vi "Receive Data From Aircraft.vi"(8 "error in (no error)":errorcluster) -> (0 "error out":errorcluster)   [LabVIEW 2014]
uses:
  Controls/Coms Driver Interface.ctl
  Telemetry/Controls/Telemetry Connection Type.ctl
  <vilib>/httpClient/ClientHandle.ctl
  Controls/Coms Driver State.ctl
  Application Support/Stop Button/SubVI/Get Stop Button Status.vi
  Web Services/DronePi Global Variables.vi
  Aircraft Information/Sub VI/Selected Aircraft/SubVI/Get Selected Aircraft.vi
  <vilib>/httpClient/LabVIEWHTTPClient.lvlib
panel:
  in  "Cluster":T1
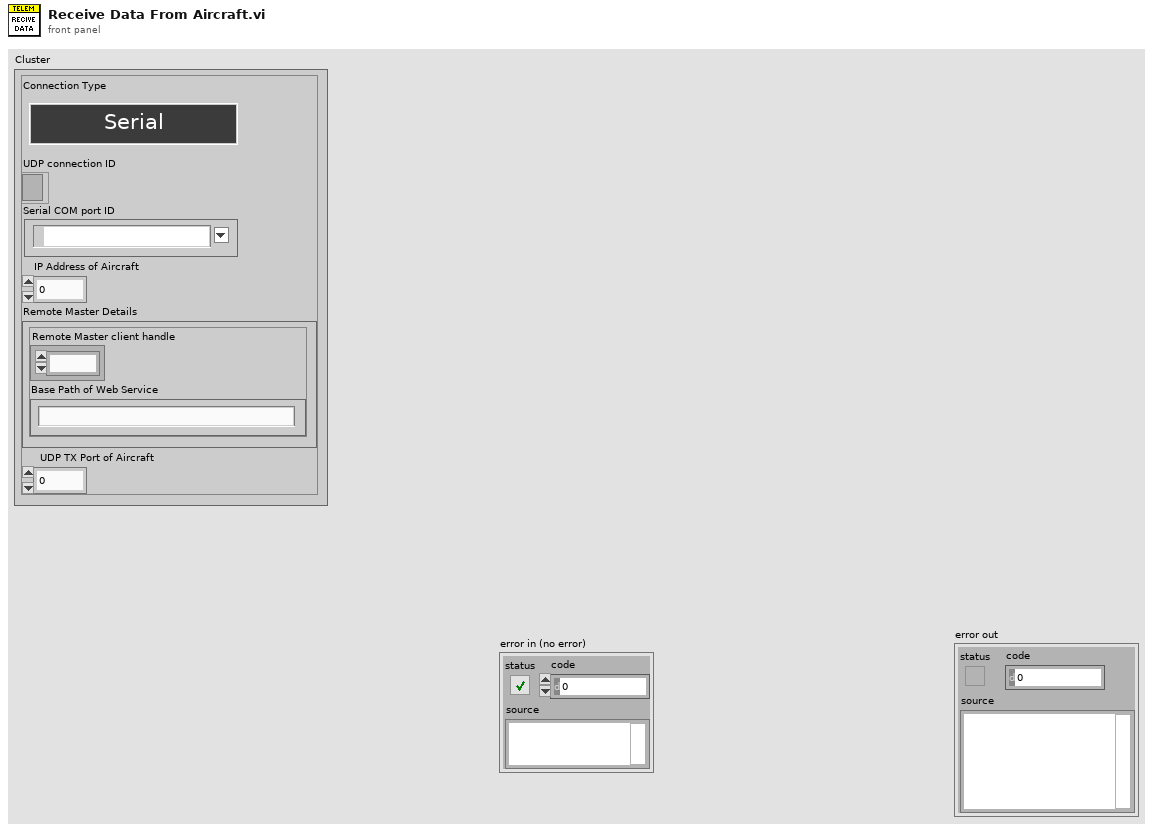
[diagram p1: front panel]
types:
  T1 = typedef "Coms Driver Interface.ctl" = cluster{"Connection Type":T2, "UDP connection ID":refnum<k16>, "Serial COM port ID":refnum<visa-resource-name>, "IP Address of Aircraft":u32, "Remote Master Details":cluster{"Remote Master client handle":T3, "Base Path of Web Service":string}, "UDP TX Port of Aircraft":u16}
  T2 = typedef "Telemetry Connection Type.ctl" = enum16{"Serial", "UDP", "Remote Master"}
  T3 = typedef "LabVIEWHTTPClient.lvlib/ClientHandle.ctl" = refnum<k1>
  T4 = typedef "Coms Driver State.ctl" = enum16{"Initalise", "Acquire Data"}
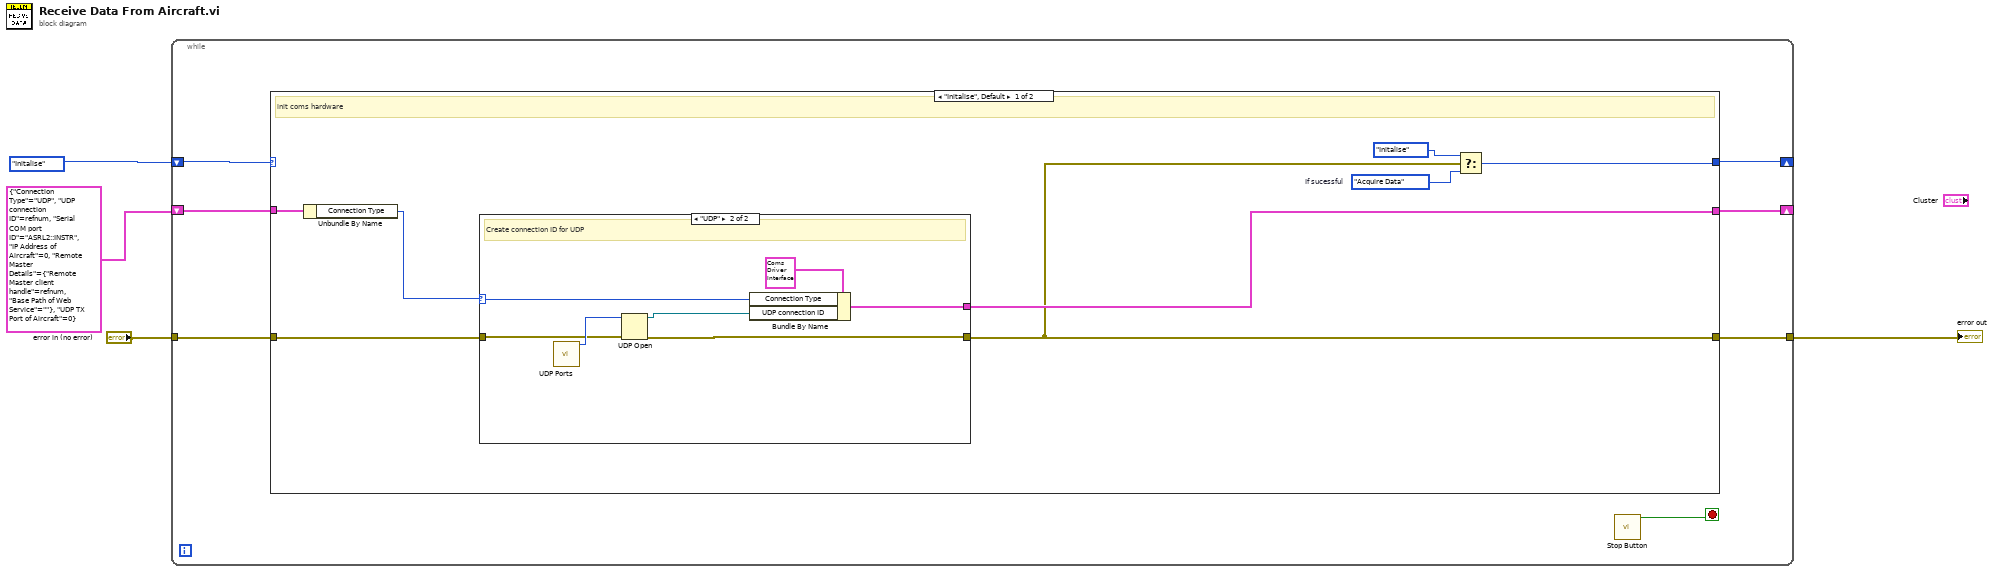
[diagram p0: block diagram]
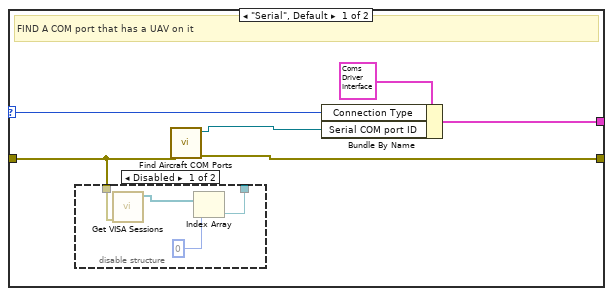
[diagram p2: hidden frame]
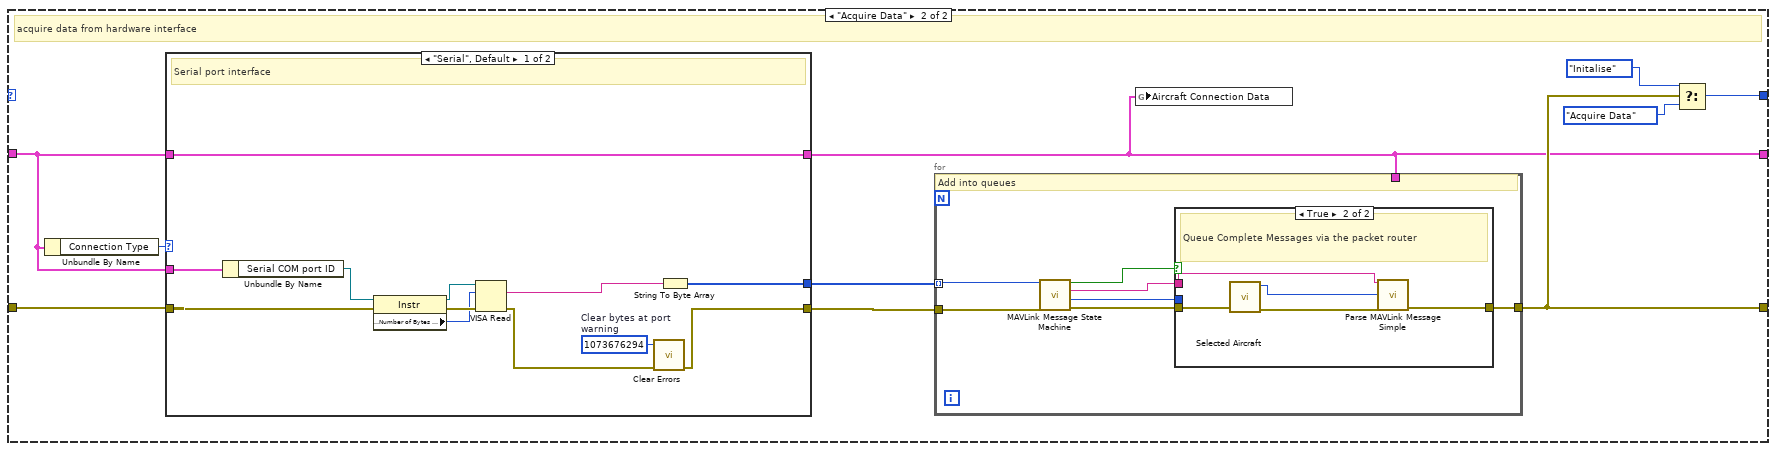
[diagram p4: hidden frame]
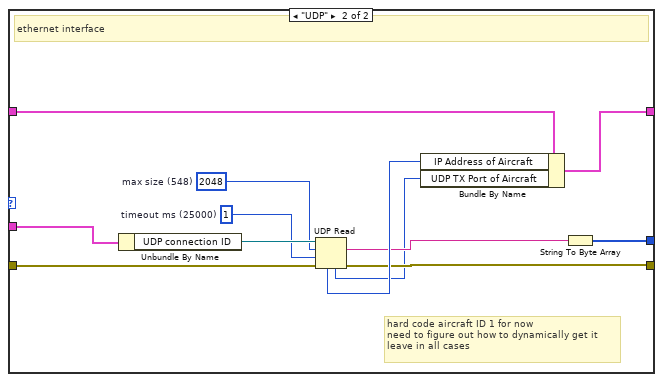
[diagram p6: hidden frame]
diagram:
  n1 = while {
    shift-right: [w7] -> _
    shift-left: Coms_Driver_State."Initalise" -> [w9]
    tunnel: "error in (no error)" -> [w11]
    tunnel: [w10] -> w3
    shift-right: [w8] -> _
    shift-left: T1 {"Connection Type"=enum."UDP", "UDP connection ID"=refnum, "Serial COM port ID"="ASRL2::INSTR", "IP Address of Aircraft"=0, "Remote Master Details"={"Remote Master client handle"=refnum, "Base Path of Web Service"=""}, "UDP TX Port of Aircraft"=0} ("Cluster") -> [w6]
    stop <- w5 stop-if-true
    n2 = case shown="\"Initalise\", Default" w9 {
      tunnel: w11 -> [w14 w44]
      tunnel: [w15 w41] -> w10
      tunnel: [w19 w37] -> w8
      tunnel: [w16 w39] -> w7
      tunnel: w6 -> [w13 w38]
      frame "Initalise", Default {
        w17 = Coms_Driver_State."Acquire Data"  # If sucessful
        # "init coms hardware"
        n3 = Unbundle By Name(w13) -> ("Connection Type"=w12:T2)
        n4 = case shown="\"UDP\"" w12 {
          selector: w12 -> [w24 w36]
          tunnel: w14 -> [w21 w31]
          tunnel: [w22 w30] -> w15
          tunnel: [w23 w34] -> w19
          frame "Serial", Default {
            # "FIND A COM port that has a UAV on it"
            n5 = disable-structure shown="Disabled" {
              disable-tunnel: w21 -> [w29 _]
              disable-tunnel: [w26 _] -> _
              frame Disabled {
                n6 = call "Get VISA Sessions.vi"("Error In"=w29) -> ("Visa Sources"=w28:refnum<visa-resource-name>[])  [unwired: 9 in, 1 out]
                n7 = Index Array(array=w28, index=0) -> (element=w26:refnum<visa-resource-name>)
              }
              frame Enabled {
              }
            }
            n8 = call "Find Aircraft COM Ports.vi"("Error In"=w21) -> ("Error Out"=w22:errorcluster, "Aircraft COM Port"=w20:refnum<visa-resource-name>)  [unwired: 9 in]
            n9 = Bundle By Name(cluster=T1 {"Connection Type"=enum."Serial", "UDP connection ID"=refnum, "Serial COM port ID"="", "IP Address of Aircraft"=0, "Remote Master Details"={"Remote Master client handle"=refnum, "Base Path of Web Service"=""}, "UDP TX Port of Aircraft"=0} ("Cluster"), "Connection Type"=w24, "Serial COM port ID"=w20) -> (w23:T1)
          }
          frame "UDP" {
            # "Create connection ID for UDP"
            n10 = call "UDP Ports.vi"() -> ("RX Port"=w33:u16)  [unwired: 9 in, 2 out]
            n11 = UDP Open(8:w31, 11:w33) -> (port=w32:refnum<k16>, 0:w30:errorcluster)  [unwired: 3 in, 1 out]
            n12 = Bundle By Name(cluster=T1 {"Connection Type"=enum."Serial", "UDP connection ID"=refnum, "Serial COM port ID"="", "IP Address of Aircraft"=0, "Remote Master Details"={"Remote Master client handle"=refnum, "Base Path of Web Service"=""}, "UDP TX Port of Aircraft"=0} ("Cluster"), "Connection Type"=w36, "UDP connection ID"=w32) -> (w34:T1)
          }
        }
        n13 = Select(t=Coms_Driver_State."Initalise", s=w15, f=w17) -> (s? t:f=w16:T4)
      }
      frame "Acquire Data" {
        # "acquire data from hardware interface"
        n14 = Unbundle By Name(w38) -> ("Connection Type"=w43:T2)
        n15 = case shown="\"Serial\", Default" w43 {
          tunnel: [w63 w74] -> w45
          tunnel: w44 -> [w67 w82]
          tunnel: [w62 w79] -> w46
          tunnel: w38 -> [w61 w78]
          tunnel: w38 -> [w60 w77]
          tunnel: [w60 w75] -> w37
          frame "Serial", Default {
            w65 = 1073676294  # Clear bytes at port warning
            # "Serial port interface"
            n16 = Unbundle By Name(w61) -> ("Serial COM port ID"=w68:refnum<visa-resource-name>)
            n17 = property class="Instr"(reference=w68, error in=w67) -> (reference out=w71:refnum<visa-resource-name>, error out=w70:errorcluster, "Serial Settings:Number of Bytes at Serial Port"=w69:u32)
            n18 = VISA Read(VISA resource name=w71, byte count=w69, error in (no error)=w70) -> (read buffer=w66:string, error out=w64:errorcluster)  [unwired: 2 out]
            n19 = call <vilib>:"Clear Errors.vi"("error in (no error)"=w64, "specific error code to clear (0: all)"=w65) -> ("error out"=w63:errorcluster)  [unwired: 4 in, 1 out]
            n20 = String To Byte Array(string=w66) -> (unsigned byte array=w62:u8[])
          }
          frame "UDP" {
            w80 = 2048  # max size (548)
            w81 = 1  # timeout ms (25000)
            # "hard code aircraft ID 1 for now\nneed to figure out how to dynamically get it\nleave in all cases"
            # "ethernet interface"
            n21 = Unbundle By Name(w78) -> ("UDP connection ID"=w83:refnum<k16>)
            n22 = UDP Read(connection ID=w83, max size (548)=w80, timeout ms (25000)=w81, 8:w82) -> (data out=w73:string, error out=w74:errorcluster, 4:w72:u16, 6:w76:u32)  [unwired: 1 out]
            n23 = Bundle By Name(cluster=w77, "IP Address of Aircraft"=w76, "UDP TX Port of Aircraft"=w72) -> (w75:T1)
            n24 = String To Byte Array(string=w73) -> (unsigned byte array=w79:u8[])
          }
        }
        n25 = for {
          tunnel: w46 -> [w53] mode=indexing
          tunnel: [w49] -> w41
          tunnel: w45 -> [w48]
          tunnel: w37 -> [_]
          # "Add into queues"
          n26 = call "MAVLink Message State Machine.vi"("Error In"=w48, "Incoming Bytes"=w53) -> ("Error Out"=w47:errorcluster, "Aircraft ID"=w50:u8, "Message"=w51:string, "Message Complete"=w52:bool)  [unwired: 6 in]
          n27 = case shown="True" w52 {
            tunnel: w51 -> [_ w58]
            tunnel: w50 -> [_ _]
            tunnel: [w54 w59] -> w49
            tunnel: w47 -> [w54 w57]
            frame False {
              # "Wait For complete message"
            }
            frame True {
              # "Queue Complete Messages via the packet router"
              n28 = call-poly "Selected Aircraft.vi"("Error In"=w57) -> ("Error Out"=w56:errorcluster, "Selected Aircraft ID Out"=w55:u8)  [unwired: 9 in]
              n29 = call "Parse MAVLink Message Simple.vi"("error in (no error)"=w56, "Aircraft ID"=w55, "Mavlink Message"=w58) -> ("error in (no error) 2"=w59:errorcluster)  [unwired: 8 in]
            }
          }
        }
        n30 = global write "DronePi Global Variables.vi" "Aircraft Connection Data"(w37) -> ()
        n31 = Select(t=Coms_Driver_State."Initalise" ("If sucessful"), s=w41, f=Coms_Driver_State."Acquire Data") -> (s? t:f=w39:T4)
      }
    }
    n32 = call-poly "Stop Button.vi"() -> ("Stop ButtonOut"=w5:bool)  [unwired: 10 in, 1 out]
  }
  "error out" <- w3
